vi "Write Limit Volt.vi"(8 "error in":errorcluster, 10 "OverVoltage_Protect":dbl, 11 "69X_79X in":refnum<class "69X_79X.lvclass">) -> (0 "error out":errorcluster, 3 "69X_79X out":refnum<class "69X_79X.lvclass">)   [LabVIEW 2019, in "69X_79X.lvlib" / "69X_79X.lvclass"]
uses:
  Library/69X_79X.lvclass
  C:/Users/Public/Documents/Development/builds/Instruments/PowerSupply.lvlibp/Library/PowerSupply.lvclass
  builds/Instruments/PowerSupply.lvlibp/Library/PowerSupply.lvclass
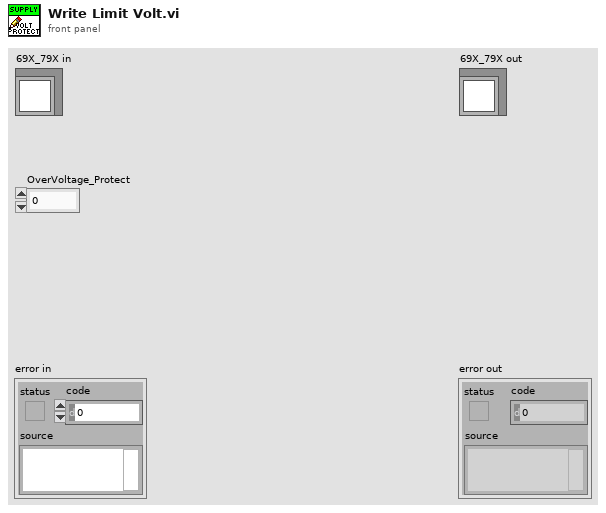
[diagram p1: front panel]
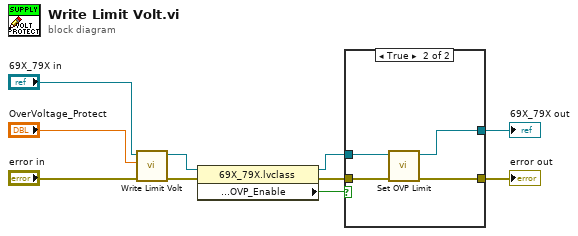
[diagram p0: block diagram]
diagram:
  n1 = call-parent "Write Limit Volt.vi"("error in"="error in", "OverVoltage_Protect"="OverVoltage_Protect", "PowerSupply in"="69X_79X in") -> ("error out"=w6:errorcluster, "PowerSupply out"=w7:refnum<class "69X_79X.lvclass">)  [unwired: 7 in]
  n2 = property class="69X_79X.lvclass"(reference=w7, error in=w6) -> (reference out=w3:refnum<class "69X_79X.lvclass">, error out=w4:errorcluster, "Accessors:Setting:Protection:OVP_Enable"=w5:bool)
  n3 = case shown="True" w5 {
    tunnel: w4 -> [w11 w16]
    tunnel: w3 -> [w12 w15]
    tunnel: [w12 w14] -> w2
    tunnel: [w11 w13] -> w1
    frame False {
    }
    frame True {
      n4 = call "Set OVP Limit.vi"("error in"=w16, "69X_79X in"=w15) -> ("error out"=w13:errorcluster, "69X_79X out"=w14:refnum<class "69X_79X.lvclass">)  [unwired: 8 in]
    }
  }
  "error out" <- w1
  "69X_79X out" <- w2
